vi "Get Data Variant.vi"(8 "error in (no error)":errorcluster, 11 "Core Groups Configuration in":refnum<class "Core Group Configuration.lvclass">) -> (0 "error out":errorcluster, 1 "data version":T1, 2 "data":variant, 3 "Core Groups Configuration out":refnum<class "Core Group Configuration.lvclass">)   [LabVIEW 2017, in "DSF Core.lvlib" / "Core Group Configuration.lvclass"]
uses:
  Core Group Configuration.lvclass
  Typedefs/DSF Version Info.ctl
  Core Group Configuration.lvclass/Core Group Configuration.ctl
  DSF Core.lvlib
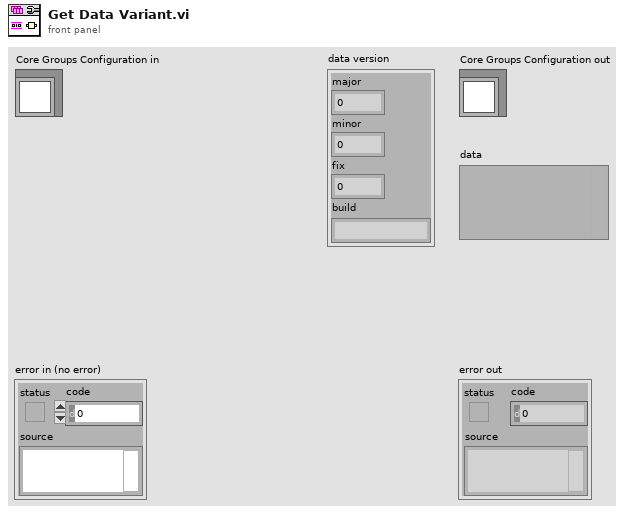
[diagram p1: front panel]
types:
  T1 = typedef "DSF Core.lvlib/DSF Version Info.ctl" = cluster{"major":u32, "minor":u32, "fix":u32, "build":string}
  T2 = typedef "DSF Core.lvlib/DSF Core Group Configuration.ctl" = cluster{"name":string, "direction":T3, "cycle timing":T4, "timeout behavior":T5}
  T3 = typedef "DSF Core.lvlib/DSF Direction.ctl" = enum8{"Tx", "Rx"}
  T4 = typedef "DSF Core.lvlib/DSF Timing Info.ctl" = cluster{"priority":u64, "decimation":u64, "offset":u64}
  T5 = typedef "DSF Core.lvlib/DSF Timeout Behavior.ctl" = enum8{"Increment Late Count", "Throw Error"}
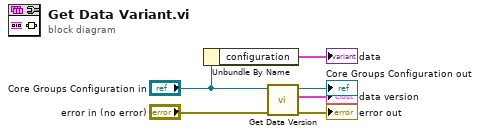
[diagram p0: block diagram]
diagram:
  n1 = Unbundle By Name("Core Groups Configuration in") -> ("configuration"=→"data":T2)
  n2 = call-dynamic "Get Data Version.vi"("error in (no error)"="error in (no error)", "Core Groups Configuration in"="Core Groups Configuration in") -> ("error out"=→"error out":errorcluster, "data version"=→"data version":T1, "Core Groups Configuration out"=→"Core Groups Configuration out":refnum<class "Core Group Configuration.lvclass">)  [unwired: 7 in]
